vi "command eesave settings.vi"(8 "error in (no error)":errorcluster, 11 "id":i32) -> (0 "error out":errorcluster, 3 "function return":i32)   [LabVIEW 2012, in "libximc.lvlib"]
doc: "result_t XIMC_API command_eesave_settings (device_t id);"
uses:
  libximc.lvlib
  libximc.dll
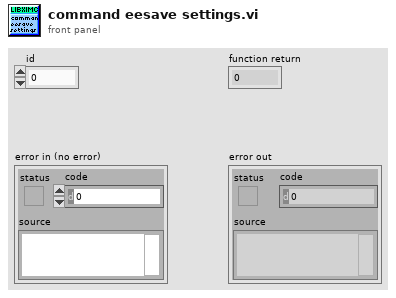
[diagram p1: front panel]
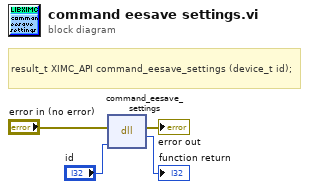
[diagram p0: block diagram]
diagram:
  # "result_t XIMC_API command_eesave_settings (device_t id);"
  n1 = dll-call lib="C:/Users/user/Desktop/labview-2.9.11-gen/libximc.*" fn="command_eesave_settings"(error in="error in (no error)", "id"="id") -> (error out=→"error out":errorcluster, →"function return":i32)  [unwired: 3 in, 1 out]
